vi "FindVar.vi"(6 "Write?":bool, 7 "Abs_Type":refnum<class "Abs_Type.lvclass">, 8 "error in (no error)":errorcluster, 9 "Tag":string, 10 "Abs_Type Default":refnum<class "Abs_Type.lvclass">, 11 "Var Bus in":refnum<class "Omni_Bus.lvclass">) -> (0 "error out":errorcluster, 1 "Updated Tag":bool, 2 "Abs_Type Found":refnum<class "Abs_Type.lvclass">, 3 "Var Bus out":refnum<class "Omni_Bus.lvclass">)   [LabVIEW 2021, in "Omni_Bus.lvclass"]
uses:
  Omni_Bus.lvclass
  <vilib>/TSA/Abstract Data Classes/Abs_Types/Type/Abs_Type.lvclass
  <vilib>/TSA/Abstract Data Classes/Abs_Types/Type/Abs_Type.lvclass/Abs_Type.ctl
  Omni_Bus.lvclass/Omni_Bus.ctl
  <vilib>/TSA/Abstract Data Classes/Abs_Types/Value/Abs_Value.lvclass
  C:/Program Files (x86)/National Instruments/LabVIEW 2021/vi.lib/TSA/Abstract Data Classes/Abs_Types/Type/Abs_Type.lvclass
  Properties/Read Var Map.vi
panel:
  # "can only be \ntrue if a value type"
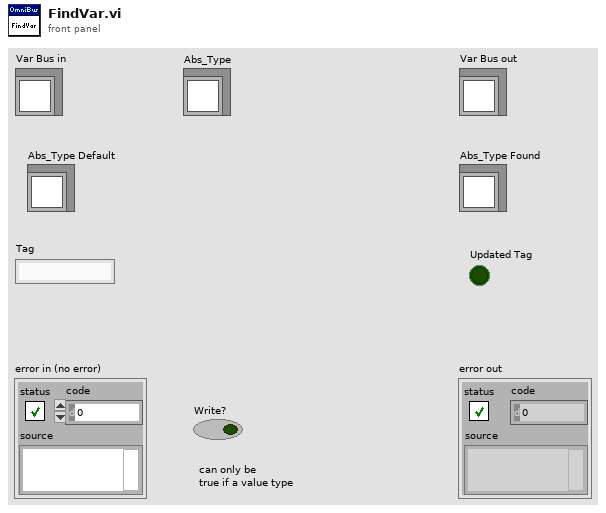
[diagram p1: front panel]
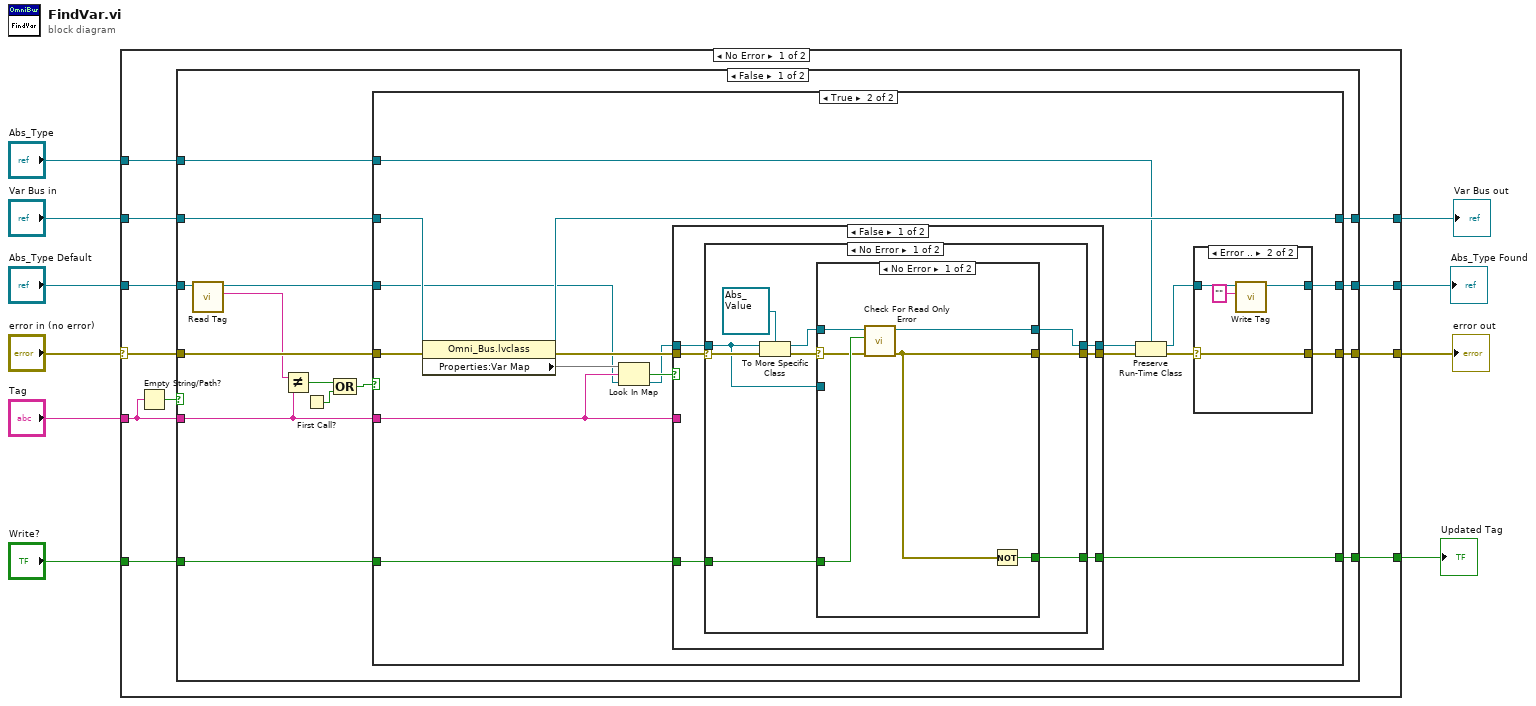
[diagram p0: block diagram]
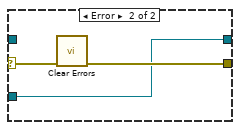
[diagram p4: hidden frame]
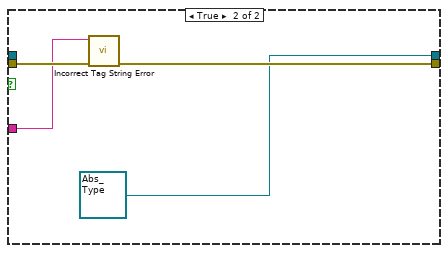
[diagram p6: hidden frame]
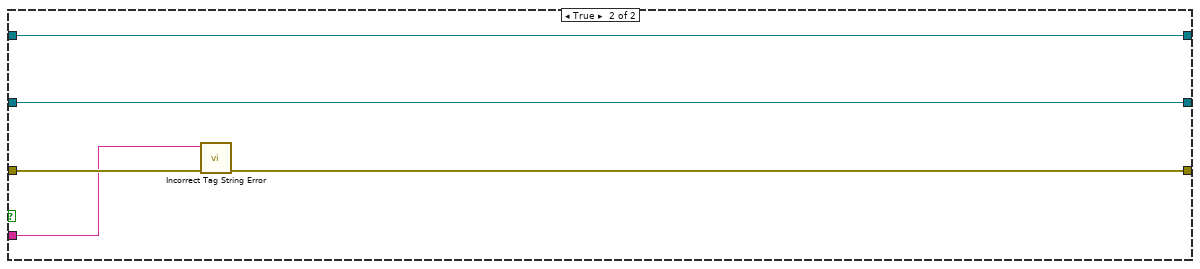
[diagram p7: hidden frame]
diagram:
  n1 = case shown="No Error" "error in (no error)" {
    selector: "error in (no error)" -> [w21 w101]
    tunnel: [w19 w101] -> w9
    tunnel: [w18 w100] -> w7
    tunnel: "Var Bus in" -> [w20 w100]
    tunnel: "Tag" -> [w16 _]
    tunnel: [w12 w99] -> w5
    tunnel: "Abs_Type Default" -> [w17 w99]
    tunnel: "Write?" -> [w14 _]
    tunnel: [w13 _] -> w2
    tunnel: "Abs_Type" -> [w11 _]
    frame No Error {
      n2 = Empty String/Path?(string/path=w16) -> (empty?=w15:bool)
      n3 = case shown="False" w15 {
        tunnel: w21 -> [w36 w97]
        tunnel: w20 -> [w35 w98]
        tunnel: [w23 w94] -> w12
        tunnel: [w34 w96] -> w19
        tunnel: [w33 w98] -> w18
        tunnel: w16 -> [w29 w95]
        tunnel: w17 -> [w28 w94]
        tunnel: w14 -> [w25 _]
        tunnel: [w24 _] -> w13
        tunnel: w11 -> [w22 _]
        frame False {
          n4 = call <vilib>:"Read Tag.vi"("Abs_Type in"=w28) -> ("Tag"=w26:string, "Abs_Type out"=w27:refnum<class "Abs_Type.lvclass">)  [unwired: 9 in]
          n5 = Not Equal?(x=w26, y=w29) -> (x != y?=w32:bool)
          n6 = First Call?() -> (First Call?: T/F=w30:bool)
          n7 = Compound Arithmetic op=OR(w32, w30) -> (w31:bool)
          n8 = case shown="True" w31 {
            tunnel: w36 -> [w38 w57]
            tunnel: w35 -> [w37 w56]
            tunnel: [w39 w41] -> w23
            tunnel: [w38 w43] -> w34
            tunnel: [w37 w54] -> w33
            tunnel: w27 -> [w39 w40]
            tunnel: w29 -> [_ w52]
            tunnel: w25 -> [_ w50]
            tunnel: [_ w49] -> w24
            tunnel: w22 -> [_ w45]
            frame False {
            }
            frame True {
              n9 = property class="Omni_Bus.lvclass"(reference=w56, error in=w57) -> (reference out=w54:refnum<class "Omni_Bus.lvclass">, error out=w53:errorcluster, "Properties:Var Map"=w55:map{string, refnum<class "Abs_Type.lvclass">})
              n10 = Look In Map(map=w55, key=w52, default value=w40) -> (key not found?=w51:bool, value=w48:refnum<class "Abs_Type.lvclass">)
              n11 = case shown="False" w51 {
                tunnel: w53 -> [w69 w93]
                tunnel: [w68 w92] -> w47
                tunnel: w52 -> [_ w91]
                tunnel: w48 -> [w67 _]
                tunnel: [w66 refnum<class "Abs_Type.lvclass"> refnum ("Abs_Type.lvclass")] -> w46
                tunnel: w50 -> [w65 _]
                tunnel: [w64 _] -> w49
                frame False {
                  n12 = case shown="No Error" w69 {
                    selector: w69 -> [w75 w89]
                    tunnel: [w74 w89] -> w68
                    tunnel: w67 -> [w71 w88]
                    tunnel: [w73 w88] -> w66
                    tunnel: w65 -> [w72 _]
                    tunnel: [w70 _] -> w64
                    frame No Error {
                      n13 = To More Specific Class(target class=refnum<class "Abs_Value.lvclass"> refnum ("Abs_Value.lvclass"), reference=w71, error in=w75) -> (specific class reference=w76:refnum<class "Abs_Value.lvclass">, error out=w77:errorcluster)
                      n14 = case shown="No Error" w77 {
                        selector: w77 -> [w82 w86]
                        tunnel: w76 -> [w83 _]
                        tunnel: [w79 w87] -> w74
                        tunnel: [w80 w85] -> w73
                        tunnel: w72 -> [w84 _]
                        tunnel: w71 -> [_ w85]
                        tunnel: [w81 _] -> w70
                        frame No Error {
                          n15 = call "Check For Read Only Error.vi"("error in (no error)"=w82, "Write?"=w84, "Abs_Value in"=w83) -> ("error out"=w79:errorcluster, "Abs_Value out"=w80:refnum<class "Abs_Value.lvclass">)  [unwired: 7 in]
                          n16 = Not(x=w79) -> (.not. x?=w81:bool)
                        }
                        frame Error {
                          n17 = call <vilib>:"Clear Errors.vi"("error in (no error)"=w86) -> ("error out"=w87:errorcluster)  [unwired: 5 in, 1 out]
                        }
                      }
                    }
                    frame Error {
                    }
                  }
                }
                frame True {
                  n18 = call "Incorrect Tag String Error.vi"("error in (no error)"=w93, "Tag"=w91) -> ("error out"=w92:errorcluster)  [unwired: 9 in]
                }
              }
              n19 = Preserve Run-Time Class(object in=w46, error in=w47, 2:w45) -> (object out=w42:refnum<class "Abs_Type.lvclass">, error out=w44:errorcluster)
              n20 = case shown="Error .." w44 {
                selector: w44 -> [w59 w63]
                tunnel: [w59 w63] -> w43
                tunnel: w42 -> [w58 w62]
                tunnel: [w58 w61] -> w41
                frame No Error {
                }
                frame Error {
                  n21 = call <vilib>:"Write Tag.vi"("Tag"="", "Abs_Type in"=w62) -> ("Abs_Type out"=w61:refnum<class "Abs_Type.lvclass">)  [unwired: 9 in]
                }
              }
            }
          }
        }
        frame True {
          n22 = call "Incorrect Tag String Error.vi"("error in (no error)"=w97, "Tag"=w95) -> ("error out"=w96:errorcluster)  [unwired: 9 in]
        }
      }
    }
    frame Error {
    }
  }
  "error out" <- w9
  "Var Bus out" <- w7
  "Abs_Type Found" <- w5
  "Updated Tag" <- w2
